vi "Main.vi"(8 "error in":errorcluster, 11 "User Worker in":refnum<class "User Worker.lvclass">) -> (0 "error out":errorcluster, 3 "User Worker out":refnum<class "User Worker.lvclass">)   [LabVIEW 2018, in "User Worker.lvclass"]
doc: "The Queued Message Handler of a Worker."
uses:
  User Worker.lvclass
  D:/Program Files (x86)/National Instruments/LabVIEW 2018/vi.lib/addons/_Workers/Library/Classes/Worker/Worker.lvclass
  <vilib>/addons/_Workers/Library/Classes/Worker/Worker.lvclass/Worker.ctl
  User Worker.lvclass/User Worker.ctl
  Initialization Data.ctl
  <vilib>/addons/_Workers/Library/Classes/Worker/Worker.lvclass
panel:
  in  "按钮 2":bool
  in  "按钮":bool
  in  "Pwd":string
  in  "User":string="operator"
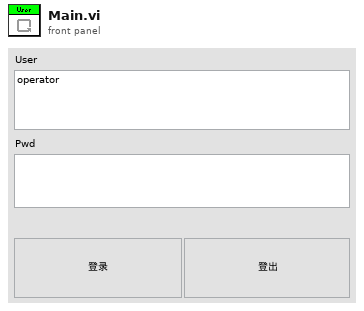
[diagram p1: front panel]
types:
  T1 = typedef "User Worker.lvclass/Initialization Data.ctl" = cluster{"String":string}
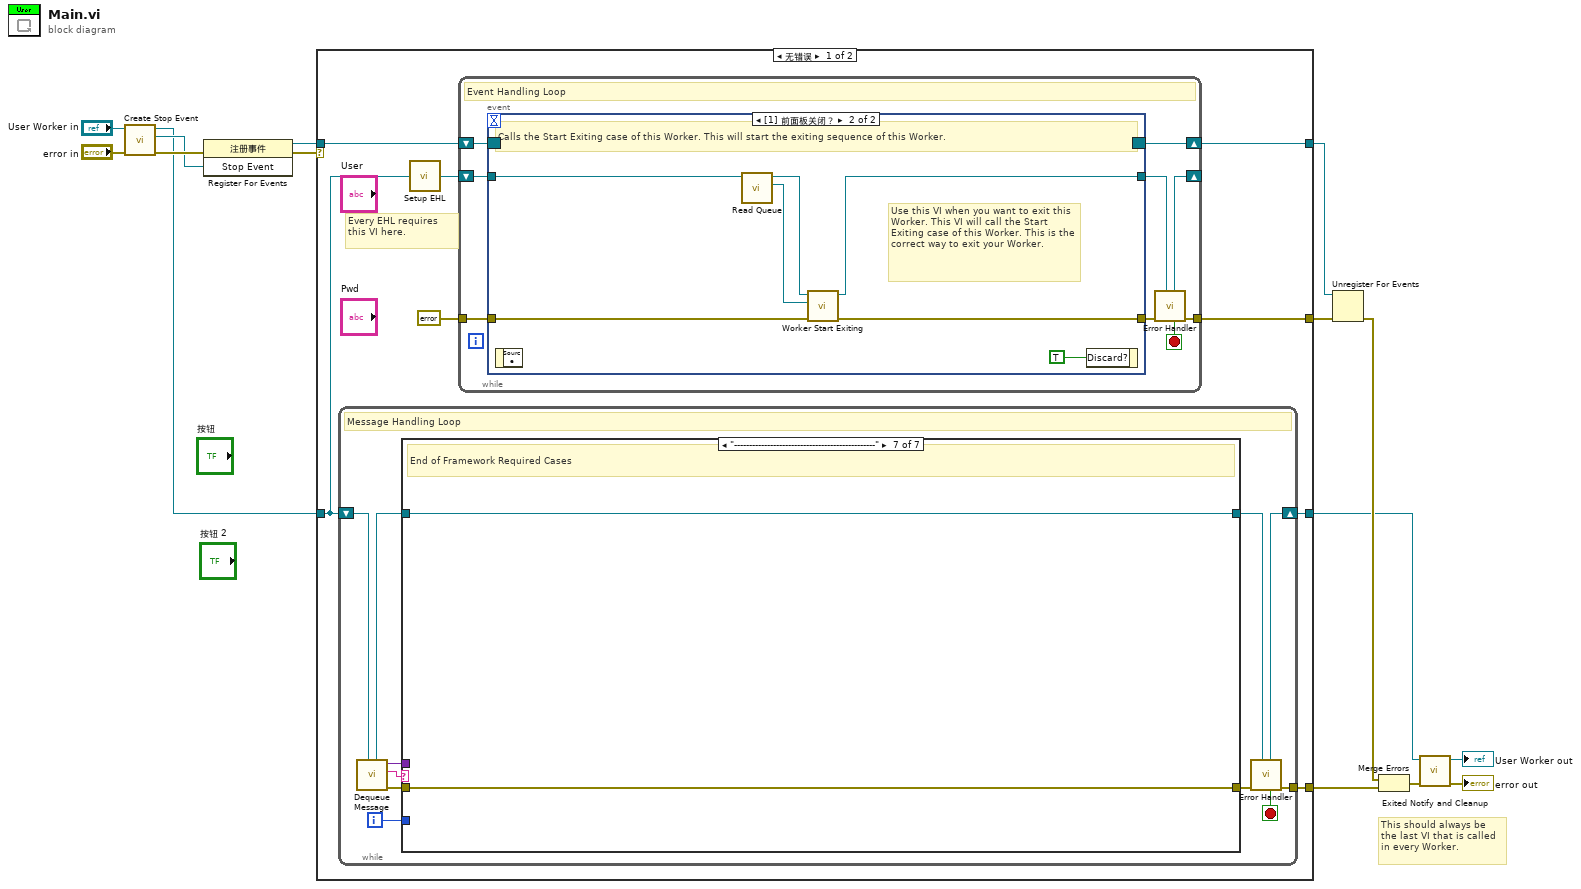
[diagram p0: block diagram]
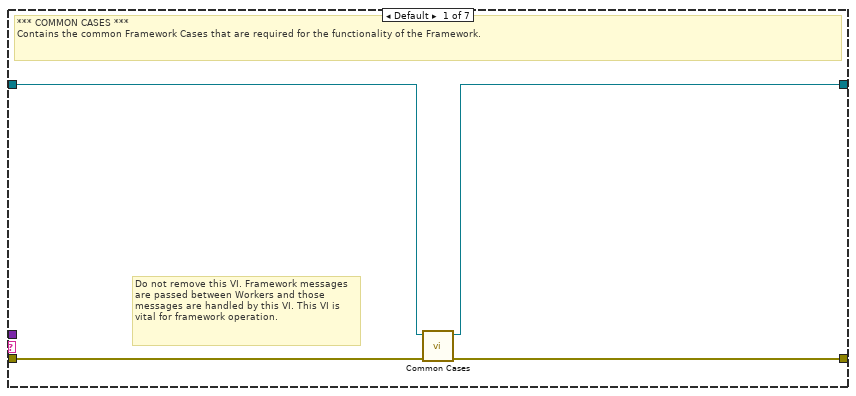
[diagram p2: hidden frame]
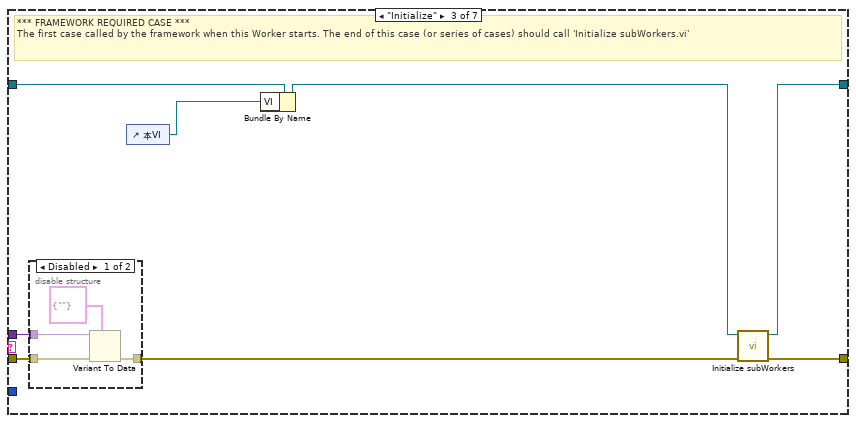
[diagram p4: hidden frame]
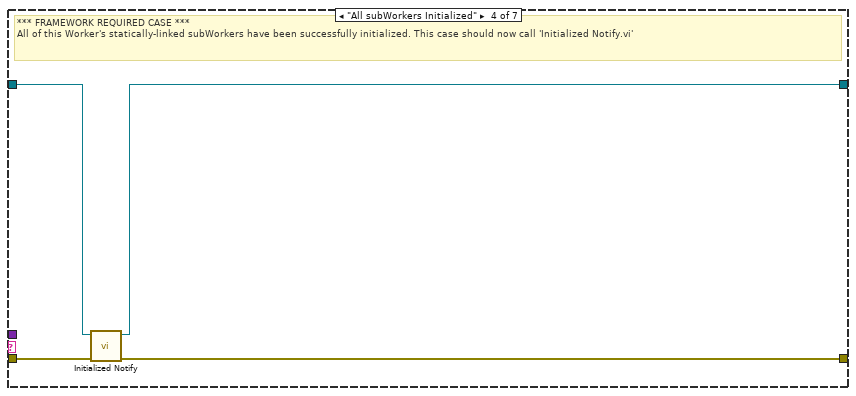
[diagram p6: hidden frame]
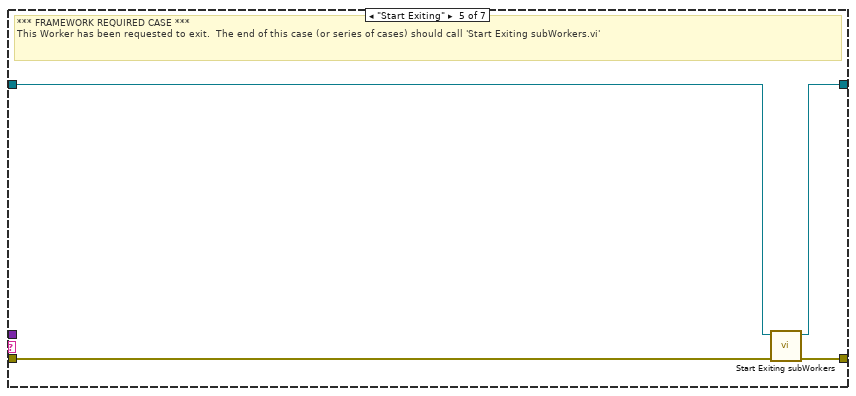
[diagram p7: hidden frame]
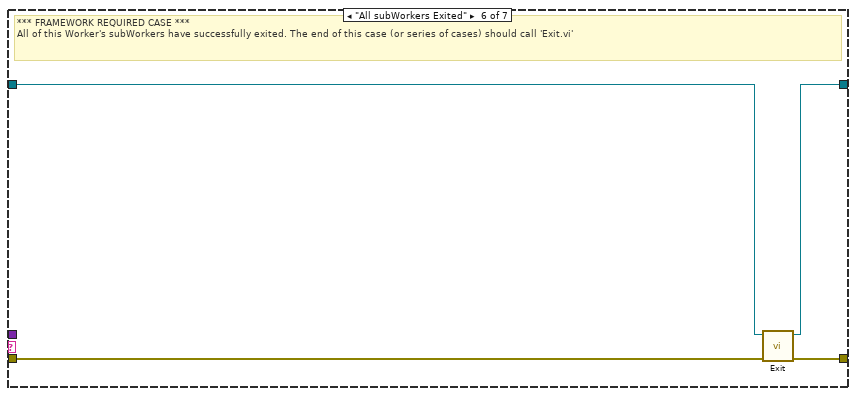
[diagram p8: hidden frame]
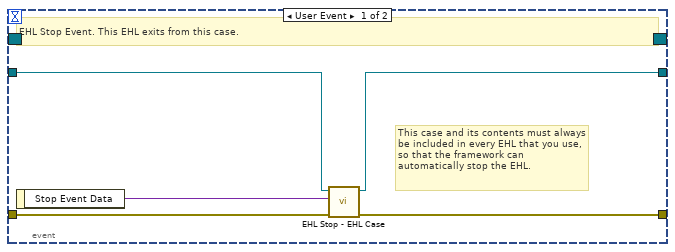
[diagram p9: hidden frame]
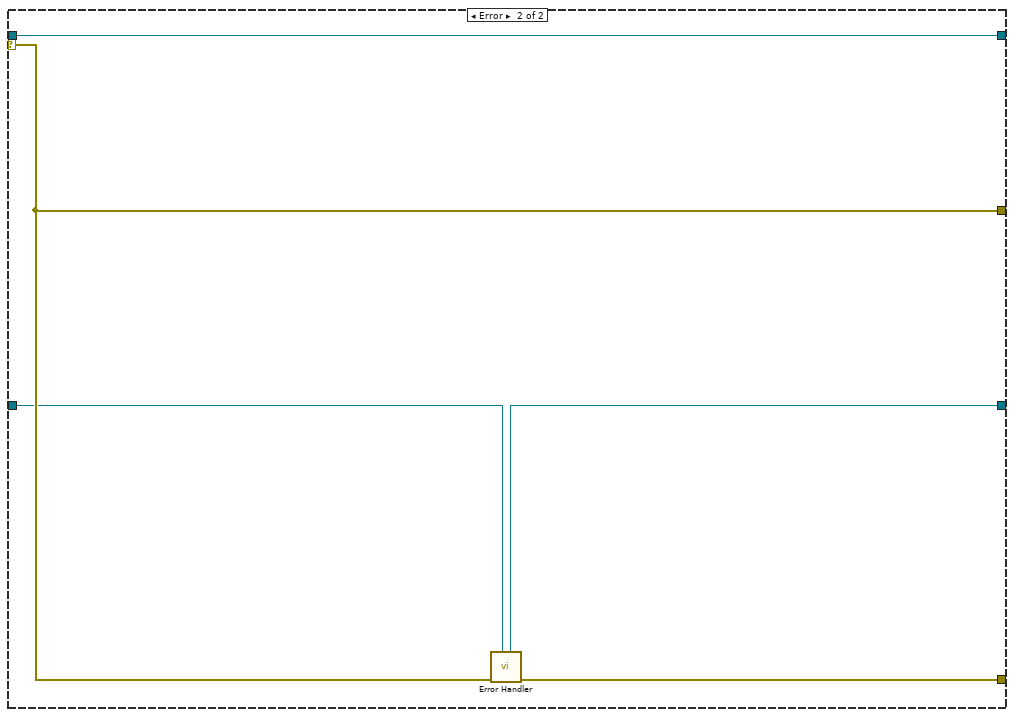
[diagram p10: hidden frame]
diagram:
  # "This should always be the last VI that is called in every Worker."
  n1 = call-dynamic "Create Stop Event.vi"("error in"="error in", "Worker"="User Worker in") -> ("error out"=w10:errorcluster, "Stop Event"=w7:refnum<user-event>, "Worker out"=w4:refnum<class "User Worker.lvclass">)  [unwired: 7 in]
  n2 = register-events(error in=w10, w7) -> (reference out=w9:refnum<event-registration>, error out=w1:errorcluster)  [unwired: 1 in]
  n3 = case shown="无错误" w1 {
    tunnel: w4 -> [w18 w90]
    tunnel: [w16 w91] -> w8
    tunnel: w9 -> [w23 w92]
    tunnel: [w20 w93] -> w14
    tunnel: [w22 w92] -> w13
    tunnel: [w17 w89] -> w11
    selector: w1 -> [_ w93]
    frame No Error {
      # "Every EHL requires\nthis VI here."
      n4 = while {
        shift-right: [w32] -> w17
        shift-left: w18 -> [w34]
        tunnel: [w33] -> w16
        i -> [w24]
        stop <- w25 stop-if-true
        # "Message Handling Loop"
        n5 = call-dynamic "Dequeue Message.vi"("Worker"=w34) -> ("error out"=w31:errorcluster, "Case out"=w26:string, "Data out"=w27:variant, "Worker out"=w29:refnum<class "User Worker.lvclass">)  [unwired: 6 in, 1 out]
        n6 = case "Worker MHL Case Structure (DO NOT CHANGE LABEL NAME)" shown="\"-----------------------------------------------\"" w26 {
          tunnel: w31 -> [w38 w39 w46 w55 w58 w65 w66]
          tunnel: [w37 w39 w48 w54 w61 w64 w66] -> w30
          tunnel: w29 -> [w36 w40 w45 w57 w59 w63 w67]
          tunnel: [w35 w40 w47 w56 w60 w62 w67] -> w28
          tunnel: w27 -> [_ _ w43 _ _ _ _]
          tunnel: w24 -> [_ _ _ _ _ _ _]
          frame Default {
            # "Do not remove this VI. Framework messages are passed between Workers and those messages are handled by this VI. This VI is vital for framework operation."
            # "*** COMMON CASES ***\nContains the common Framework Cases that are required for the functionality of the Framework."
            n7 = call-dynamic "Common Cases.vi"("error in"=w38, "Comm Worker in"=w36) -> ("error out"=w37:errorcluster, "Comm Worker out"=w35:refnum<class "User Worker.lvclass">)  [unwired: 8 in]
          }
          frame "------ FRAMEWORK REQUIRED CASES ------" {
            # "Start of Framework Required Cases"
          }
          frame "Initialize" {
            # "*** FRAMEWORK REQUIRED CASE ***\nThe first case called by the framework when this Worker starts. The end of this case (or series of cases) should call 'Initialize subWorkers.vi'"
            n8 = disable-structure shown="Disabled" {
              disable-tunnel: w46 -> [w52 w53]
              disable-tunnel: [w51 w53] -> w44
              disable-tunnel: w43 -> [w50 _]
              frame Disabled {
                n9 = Variant To Data(error in=w52, type=T1 {"String"=""} ("Initialization Data"), Variant=w50) -> (error out=w51:errorcluster)  [unwired: 1 out]
              }
              frame Enabled {
              }
            }
            n10 = control-ref of="本VI"() -> (w41:refnum<vi>)
            n11 = Bundle By Name(cluster=w45, "VI"=w41) -> (w42:refnum<class "User Worker.lvclass">)
            n12 = call-dynamic "Initialize subWorkers.vi"("error in"=w44, "Worker"=w42) -> ("error out"=w48:errorcluster, "dup Worker out"=w47:refnum<class "User Worker.lvclass">)  [unwired: 8 in]
          }
          frame "All subWorkers Initialized" {
            # "*** FRAMEWORK REQUIRED CASE ***\nAll of this Worker's statically-linked subWorkers have been successfully initialized. This case should now call 'Initialized Notify.vi'"
            n13 = call-dynamic "Initialized Notify.vi"("error in"=w55, "Worker"=w57) -> ("error out"=w54:errorcluster, "dup Worker out"=w56:refnum<class "User Worker.lvclass">)  [unwired: 8 in]
          }
          frame "Start Exiting" {
            # "*** FRAMEWORK REQUIRED CASE ***\nThis Worker has been requested to exit.  The end of this case (or series of cases) should call 'Start Exiting subWorkers.vi'"
            n14 = call-dynamic "Start Exiting subWorkers.vi"("error_in"=w58, "Worker"=w59) -> ("error out"=w61:errorcluster, "dup Worker out"=w60:refnum<class "User Worker.lvclass">)  [unwired: 8 in]
          }
          frame "All subWorkers Exited" {
            # "*** FRAMEWORK REQUIRED CASE ***\nAll of this Worker's subWorkers have successfully exited. The end of this case (or series of cases) should call 'Exit.vi'"
            n15 = call-dynamic "Exit.vi"("error_in"=w65, "Worker"=w63) -> ("error out"=w64:errorcluster, "dup Worker out"=w62:refnum<class "User Worker.lvclass">)  [unwired: 8 in]
          }
          frame "-----------------------------------------------" {
            # "End of Framework Required Cases"
          }
        }
        n16 = call-dynamic "Error Handler.vi"("Worker"=w28, "error_in"=w30) -> ("error out"=w33:errorcluster, "Stop Loop"=w25:bool, "Worker out"=w32:refnum<class "User Worker.lvclass">)  [unwired: 7 in]
      }
      n17 = call-dynamic "Setup EHL.vi"("Worker"=w18) -> ("Worker out"=w19:refnum<class "User Worker.lvclass">)  [unwired: 14 in]
      n18 = while "Event Handling Loop" {
        shift-right: [w76] -> w22
        shift-left: w23 -> [w75]
        tunnel: [w71] -> w20
        tunnel: errorcluster {"status"=FALSE, "code"=0, "source"=""} ("error constant") -> [w73]
        shift-right: [w69] -> _
        shift-left: w19 -> [w74]
        stop <- w68 stop-if-true
        # "Event Handling Loop"
        n19 = event shown="[1] 前面板关闭？" {
          selector: w75 -> [_ _]
          dyn-events: [_ _] -> w76
          timeout: _ -> [_ _]
          tunnel: [w80 w87] -> w72
          tunnel: w73 -> [w81 w86]
          tunnel: w74 -> [w79 w85]
          tunnel: [w78 w84] -> w70
          event User Event {
            # "This case and its contents must always be included in every EHL that you use, so that the framework can automatically stop the EHL."
            # "EHL Stop Event. This EHL exits from this case."
            n20 = event-data() -> ("Stop Event Data"=w77:variant)  [unwired: 1 in]
            n21 = call <vilib>:"EHL Stop - EHL Case.vi"("error in"=w81, "Stop Event Data"=w77, "Worker"=w79) -> ("error out"=w80:errorcluster, "Worker out"=w78:refnum<class "User Worker.lvclass">)  [unwired: 7 in]
          }
          event Panel Close? {
            # "Use this VI when you want to exit this Worker. This VI will call the Start Exiting case of this Worker. This is the correct way to exit your Worker."
            # "Calls the Start Exiting case of this Worker. This will start the exiting sequence of this Worker."
            n22 = event-data() -> ()  [unwired: 1 in, 1 out]
            n23 = call <vilib>:"Read Queue.vi"("Worker"=w85) -> ("Message Queue out"=w82:refnum<class "Message Queue.lvclass">, "dup Worker out"=w83:refnum<class "User Worker.lvclass">)  [unwired: 9 in]
            n24 = call-dynamic "Worker Start Exiting.vi"("error_in"=w86, "Message Queue"=w82, "Worker"=w83) -> ("error out"=w87:errorcluster, "dup Worker out"=w84:refnum<class "User Worker.lvclass">)  [unwired: 7 in]
            n25 = event-data("Discard?"=TRUE) -> ()  [unwired: 1 in, 1 out]
          }
        }
        n26 = call-dynamic "Error Handler.vi"("Worker"=w70, "error_in"=w72) -> ("error out"=w71:errorcluster, "Stop Loop"=w68:bool, "Worker out"=w69:refnum<class "User Worker.lvclass">)  [unwired: 7 in]
      }
    }
    frame Error {
      n27 = call-dynamic "Error Handler.vi"("Worker"=w90, "error_in"=w93) -> ("error out"=w91:errorcluster, "Worker out"=w89:refnum<class "User Worker.lvclass">)  [unwired: 7 in, 1 out]
    }
  }
  n28 = Unregister For Events(event registration refnum=w13, error in=w14) -> (error out=w15:errorcluster)
  n29 = Merge Errors(w15, w8) -> (w12:errorcluster)
  n30 = call-dynamic "Exited Notify and Cleanup.vi"("error_in"=w12, "Worker"=w11) -> ("error out"=→"error out":errorcluster, "dup Worker out"=→"User Worker out":refnum<class "User Worker.lvclass">)  [unwired: 8 in]
